vi "Clusterwitharraytextring.vi"(1 "Cluster In":cluster{"Array In":u16[], "Ring":u16} {"Ring" items=["hello", "there"]; "Array In" items=["hello", "there"]}) -> (0 "Cluster Out":cluster{"Array Out":u16[], "Ring":u16} {"Ring" items=["hello", "there"]; "Array Out" items=["hello", "there"]})   [LabVIEW 2012]
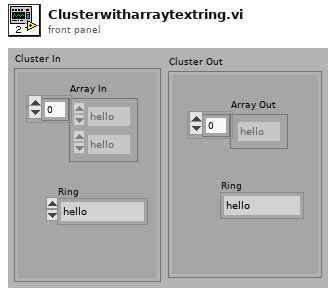
[diagram p1: front panel]
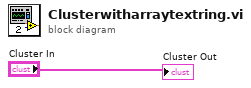
[diagram p0: block diagram]
diagram:
  "Cluster Out" <- "Cluster In"
